vi "NotchCoeffMultiChanTemplate.vi"(0 "notch frequency":dbl=2.0 format="%#_6p", 5 "notch width":dbl=20.0 format="%#_6p", 9 "sample rate":dbl=50000.0 format="%#_6p", 11 "error in (no error)":errorcluster, 12 "channel index":u16) -> (4 "configuration":T1, 15 "error out":errorcluster)   [LabVIEW 2017, in "NI_FpgaMspHost.lvlib"]
doc: "This VI designs a Butterworth filter, then quantizes and formats the coefficients into 32-bit integers for use by the Butterworth Filter VI on the FPGA.\n\nThe user is responsible for ensuring that the configuration is valid. The following restrictions apply:\nCutoff frequency must meet Nyquist criterion.\nMultichannel filters are restricted to 2nd order.\nFilter order and type cannot be changed at run-time."
uses:
  <vilib>/rvi/Analysis/host/Public/NI_FpgaMspHost.lvlib
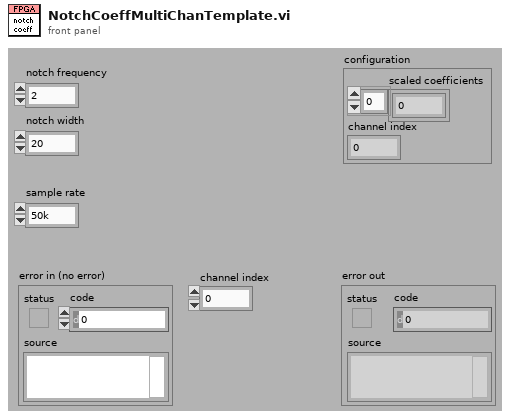
[diagram p1: front panel]
types:
  T1 = cluster{"scaled coefficients":i32[], "channel index":u16}
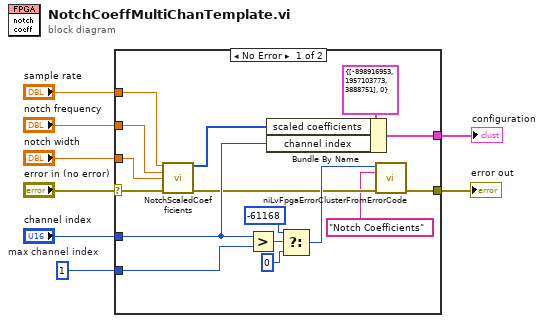
[diagram p0: block diagram]
diagram:
  w3 = u16 1  # max channel index
  n1 = case shown="No Error" "error in (no error)" {
    selector: "error in (no error)" -> [w13 w25]
    tunnel: [w10 w25] -> w8
    tunnel: "sample rate" -> [w24 _]
    tunnel: "notch frequency" -> [w23 _]
    tunnel: [w20 _] -> w5
    tunnel: "notch width" -> [w19 _]
    tunnel: w3 -> [w15 _]
    tunnel: "channel index" -> [w14 _]
    frame No Error {
      n2 = call <vilib>:"NotchScaledCoefficients.vi"("sample rate (S/s)"=w24, "notch frequency (Hz)"=w23, "notch width (Hz)"=w19, "error in (no error)"=w13) -> ("scaled coefficients"=w21:i32[], "error out"=w11:errorcluster)  [unwired: 2 in, 8 out]
      n3 = Greater?(x=w14, y=w15) -> (0:w18:bool)
      n4 = Bundle By Name(cluster=T1 {"scaled coefficients"=[-898916953, 1957103773, 3888751], "channel index"=0} ("scaled coefficients"), "scaled coefficients"=w21, "channel index"=w14) -> (w20:T1)
      n5 = Select(t=-61168, s=w18, f=0 ("Error Code")) -> (s? t:f=w12:i32)
      n6 = call <vilib>:"niLvFpgaErrorClusterFromErrorCode.vi"("error code"=w12, "function name"="Notch Coefficients" ("subVI name"), "error in"=w11) -> ("error out"=w10:errorcluster)  [unwired: 4 in, 8 out]
    }
    frame Error {
    }
  }
  "error out" <- w8
  "configuration" <- w5
